vi "CODMn通讯.vi"() -> ()   [LabVIEW 2016, in "斯坦道CODMn新电路板.lvlib"]
uses:
  <vilib>/NI/Modbus Library/API/Wrapper/Create TCP Slave.vi
  <vilib>/Utility/config.llb/Write Key (String).vi
  <vilib>/Plasmionique/MB Master/MB_Master/MB_Master.lvclass
  <vilib>/NI/Modbus Library/API/slave/Modbus Slave.lvclass
  <vilib>/Utility/config.llb/NI_LVConfig.lvlib
  <vilib>/Plasmionique/MB Master/MB Master.lvlib
  <vilib>/NI/Modbus Library/API/Wrapper/API Main.lvlib
  Alarm interface/Alarm interface.lvlib
  <vilib>/ptbypt/NI_PtbyPt.lvlib
panel:
  out "控制命令 2":u16[](array[numeric]) format="%xH"
  out "状态告警区":T1 {"工作状态" items=["空闲"=0, "水样测试"=1, "标样核查"=2, "零点核查"=3, "跨度核查"=4, "空白测试"=5, "平行样测试"=6, "加标回收"=7, "空白校准"=8, "标样校准"=9, "初始化（清洗）"=10, "调试"=22, "填充管路"=30, "清洗管路"=31, "清洗反应杯"=32]; "告警代码" items=["无告警", "缺试剂告警", "缺水样告警", "缺蒸馏水告警", "缺标液告警", "仪表漏液告警", "标定异常告警", "超量程告警", "加热异常", "低试剂预警", "超上限告警", "超下限告警", "仪表内部其他异常", "滴定异常告警", "电极异常告警", "量程切换告警", "参数设置告警", "PH电极电位异常", "电导率电极异常", "浊度光度异常", "溶解氧电极异常", "溶解氧光强异常", "温度异常告警", "PH异常告警", "溶解氧异常告警", "电导率异常告警", "浊度异常告警", "叶绿素异常告警", "藻密度异常告警", "蓝绿藻异常告警", "ORP异常告警", "氨氮异常告警", "清洁刷异常告警", "SD卡异常告警", "蓝牙异常告警", "Wifi异常告警", "流程异常告警"]; "故障代码" items=["无故障", "电机故障", "温度故障", "通讯故障", "滴定故障"]}
  out "测量数据区":T2 {"单位" items=["ug/L", "mg/L", "ppm", "mg/m3", "cm", "ppb", "ug/m3", "%", "nmol/mol", "umol/mol", "MPN/L", "MPN/100ml", "ng/m3", "NTU", "无量纲", "ms/cm", "us/cm", "℃", "mV", "万个/L"]}
  out "状态告警区":u16[](array[numeric])
  out "测量数据区":u16[](array[numeric])
  out "序列号":string
  out "status":bool
  out "关键参数区":T3
  in  "读关键参数区":bool
  in  "读状态告警区":bool
  in  "读测量数据区":bool
  in  "站号":u16(ring) items=["CODMn"=21, "氨氮"=3]
  in  "停止":bool
  in  "启动":bool
  in  "控制命令":u16(ring) items=["启动测量"=1, "标样核查"=2, "零点核查"=3, "跨度核查"=4, "空白测试"=5, "平行样测试"=6, "加标回收"=7, "空白校准"=8, "标样校准"=9, "初始化（清洗）"=10, "停止测试"=11, "仪器重启"=12, "校时"=13, "模式设置"=14, "测量间隔设置"=15]
  in  "控制命令参数":u16[](array[numeric]) format="%04xH"
  in  "VISA Resource":refnum<visa-resource-name>
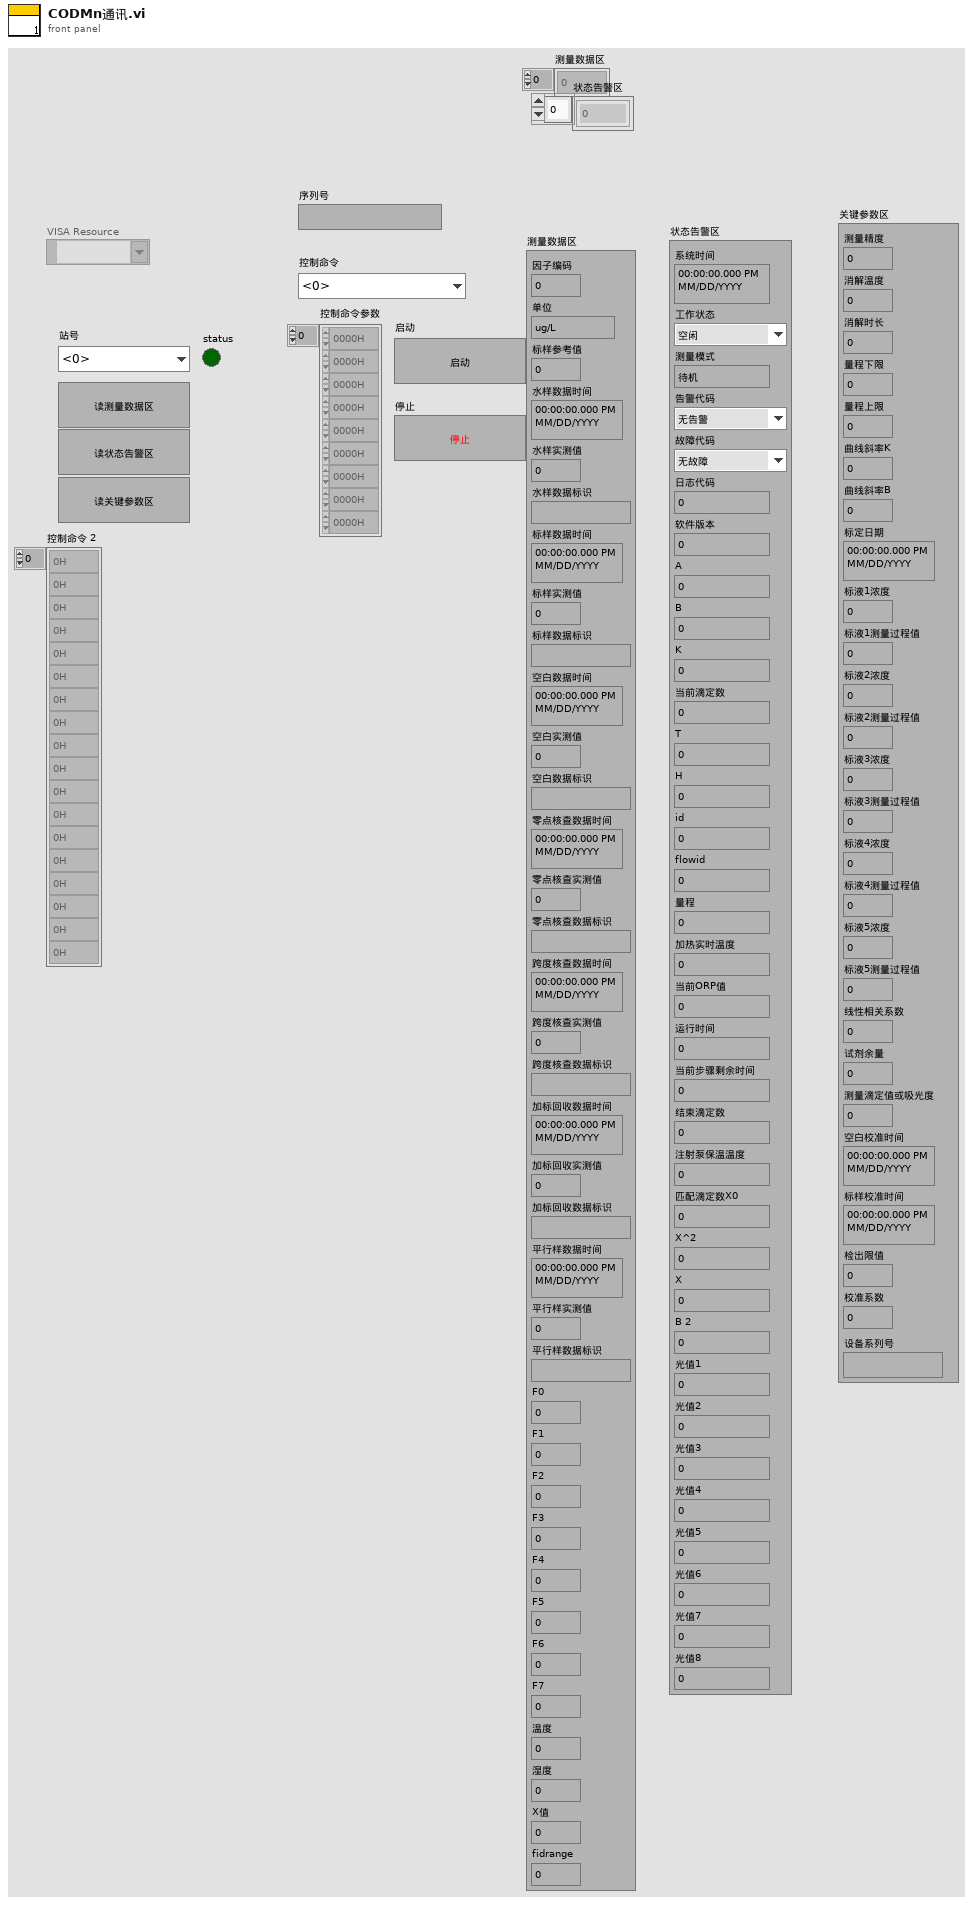
[diagram p1: front panel]
types:
  T1 = cluster{"系统时间":timestamp, "工作状态":u16, "测量模式":enum16{"待机", "连续模式", "周期模式", "定点模式", "受控模式", "手动模式"}, "告警代码":u16, "故障代码":u16, "日志代码":u16, "软件版本":u16, "A":sgl, "B":sgl, "K":sgl, "当前滴定数":sgl, "T":sgl, "H":sgl, "id":u16, "flowid":u16, "量程":u16, "加热实时温度":sgl, "当前ORP值":sgl, "运行时间":sgl, "当前步骤剩余时间":sgl, "结束滴定数":sgl, "注射泵保温温度":sgl, "匹配滴定数X0":u16, "X^2":sgl, "X":sgl, "B 2":sgl, "光值1":sgl, "光值2":sgl, "光值3":sgl, "光值4":sgl, "光值5":sgl, "光值6":sgl, "光值7":sgl, "光值8":sgl}
  T2 = cluster{"因子编码":u32, "单位":u16, "标样参考值":sgl, "水样数据时间":timestamp, "水样实测值":sgl, "水样数据标识":string, "标样数据时间":timestamp, "标样实测值":sgl, "标样数据标识":string, "空白数据时间":timestamp, "空白实测值":sgl, "空白数据标识":string, "零点核查数据时间":timestamp, "零点核查实测值":sgl, "零点核查数据标识":string, "跨度核查数据时间":timestamp, "跨度核查实测值":sgl, "跨度核查数据标识":string, "加标回收数据时间":timestamp, "加标回收实测值":sgl, "加标回收数据标识":string, "平行样数据时间":timestamp, "平行样实测值":sgl, "平行样数据标识":string, "F0":sgl, "F1":sgl, "F2":sgl, "F3":sgl, "F4":sgl, "F5":sgl, "F6":sgl, "F7":sgl, "温度":sgl, "湿度":sgl, "X值":sgl, "fidrange":sgl}
  T3 = cluster{"测量精度":u16, "消解温度":u16, "消解时长":u16, "量程下限":sgl, "量程上限":sgl, "曲线斜率K":sgl, "曲线斜率B":sgl, "标定日期":timestamp, "标液1浓度":sgl, "标液1测量过程值":sgl, "标液2浓度":sgl, "标液2测量过程值":sgl, "标液3浓度":sgl, "标液3测量过程值":sgl, "标液4浓度":sgl, "标液4测量过程值":sgl, "标液5浓度":sgl, "标液5测量过程值":sgl, "线性相关系数":sgl, "试剂余量":u32, "测量滴定值或吸光度":sgl, "空白校准时间":timestamp, "标样校准时间":timestamp, "检出限值":sgl, "校准系数":sgl, "设备系列号":string}
  T4 = enum16{"", "CODMn", "PH", "氨氮", "总氮", "总磷", "CODCr", "电导率", "水温", "溶解氧", "浊度", "叶绿素", "藻密度", "ORP"}
  T5 = typedef "CODMn交互.ctl" = cluster{"COD浓度（mg/L)":dbl, "水样启动时间":timestamp, "加标回收启动时间":timestamp, "CODMn工作状态":enum16{"空闲", "水样测试", "标样核查", "零点核查", "跨度核查", "空白测试", "平行样测试", "加标回收", "空白校准", "标样校准", "初始化（清洗）"}, "多列列表框":i32, "平台试剂余量百分比":sgl, "关键参数":cluster{"测量量程":dbl, "测量精度":dbl, "测量间隔":dbl, "消解温度":dbl, "消解时长":dbl, "空白校准时间":timestamp, "曲线截距":dbl, "曲线斜率":dbl, "测量检出限":dbl, "测量信号值":dbl, "线性相关系数":dbl, "二次多项式系数":dbl, "标样校准时间":timestamp, "稀释倍数":dbl, "三项式系数":dbl, "空白标定系数":dbl, "量程系数":dbl, "F0/ORPA":dbl, "F1/ORPB":dbl, "F2/ORPK":dbl, "F3":dbl, "F4":dbl, "F5":dbl, "F6":dbl, "F7":dbl, "X0/滴定数":dbl, "量程":dbl}, "关键参数改变":bool, "校准信息":cluster{"低标液1浓度":dbl, "低标液1信号值":dbl, "低标液1启用":u16, "低标液2浓度":dbl, "低标液2信号值":dbl, "低标液2启用":u16, "低标液3浓度":dbl, "低标液3信号值":dbl, "低标液3启用":u16, "低标液4浓度":dbl, "低标液4信号值":dbl, "低标液4启用":u16, "低标液5浓度":dbl, "低标液5信号值":dbl, "低标液5启用":u16, "高标液1浓度":dbl, "高标液1信号值":dbl, "高标液1启用":u16, "高标液2浓度":dbl, "高标液2信号值":dbl, "高标液2启用":u16, "高标液3浓度":dbl, "高标液3信号值":dbl, "高标液3启用":u16, "高标液4浓度":dbl, "高标液4信号值":dbl, "高标液4启用":u16, "高标液5浓度":dbl, "高标液5信号值":dbl, "高标液5启用":u16, "低斜率":dbl, "低截距":dbl, "低二次多项式系数":dbl, "低线性相关系数":dbl, "高斜率":dbl, "高截距":dbl, "高二次多项式系数":dbl, "高线性相关系数":dbl}, "校准信息改变":bool, "固件版本号":string}
  T6 = cluster{"测量模式":enum16{"水样测量", "标样核查", "零点核查", "跨度核查", "空白测试", "加标回收", "平行样", "校零", "校标"}}
  T7 = cluster{"时间标识":timestamp, "设备":string, "日志信息":string, "流程参数":string}
  T8 = typedef "NI_LVConfig.lvlib/Config Data RefNum.ctl" = refnum<k1>
  T9 = typedef "量程选择控件.ctl" = enum32{"L", "H", "AUTO"}
  T10 = cluster{"水样测试量程模式":T9, "标样核查量程模式":T9, "零点核查量程模式":T9, "跨度核查量程模式":T9, "空白测试量程模式":T9, "平行样测试量程模式":T9, "加标回收量程模式":T9, "空白校准量程模式":T9, "标样校准量程模式":T9}
  T11 = cluster{"测量量程":dbl, "测量精度":dbl, "测量间隔":dbl, "消解温度":dbl, "消解时长":dbl, "空白校准时间":timestamp, "曲线截距":dbl, "曲线斜率":dbl, "测量检出限":dbl, "测量信号值":dbl, "线性相关系数":dbl, "二次多项式系数":dbl, "标样校准时间":timestamp, "稀释倍数":dbl, "三项式系数":dbl, "空白标定系数":dbl, "量程系数":dbl, "F0/ORPA":dbl, "F1/ORPB":dbl, "F2/ORPK":dbl, "F3":dbl, "F4":dbl, "F5":dbl, "F6":dbl, "F7":dbl, "X0/滴定数":dbl, "量程":dbl}
  T12 = cluster{"低标液1浓度":dbl, "低标液1信号值":dbl, "低标液1启用":u16, "低标液2浓度":dbl, "低标液2信号值":dbl, "低标液2启用":u16, "低标液3浓度":dbl, "低标液3信号值":dbl, "低标液3启用":u16, "低标液4浓度":dbl, "低标液4信号值":dbl, "低标液4启用":u16, "低标液5浓度":dbl, "低标液5信号值":dbl, "低标液5启用":u16, "高标液1浓度":dbl, "高标液1信号值":dbl, "高标液1启用":u16, "高标液2浓度":dbl, "高标液2信号值":dbl, "高标液2启用":u16, "高标液3浓度":dbl, "高标液3信号值":dbl, "高标液3启用":u16, "高标液4浓度":dbl, "高标液4信号值":dbl, "高标液4启用":u16, "高标液5浓度":dbl, "高标液5信号值":dbl, "高标液5启用":u16, "低斜率":dbl, "低截距":dbl, "低二次多项式系数":dbl, "低线性相关系数":dbl, "高斜率":dbl, "高截距":dbl, "高二次多项式系数":dbl, "高线性相关系数":dbl}
  T13 = cluster{"站号":u16, "量程切换":enum32{"H", "L", "AUTO"}, "控制命令":u16, "模式设置":enum16{"待机", "连续模式", "周期模式", "定点模式", "受控模式", "手动模式"}, "测量间隔":u16}
  T14 = enum16{"水样测量", "标样核查", "零点核查", "跨度核查", "空白测试", "加标回收", "平行样", "校零", "校标"}
  T15 = enum8{"Enabled", "Disabled", "Disabled and Grayed Out"}
  T16 = typedef "Alarm interface.lvlib/map in.ctl" = cluster{"name":string, "CN":string, "FirmwareVersion":string, "code":string}
  T17 = typedef "工况数据.ctl" = cluster{"time":string, "data":cluster{"ups":cluster{"ups":cluster{"input_voltage":ext, "input_frequency":ext, "output_voltage":ext, "output_current":ext, "output_frequency":ext, "output_active_power":ext, "output_apparent_power":ext, "load_rate":ext, "cabinet_temperature":ext, "battery_voltage":ext, "remaining_battery_capacity":ext, "power_on_status":string, "power_supply_mode":string, "fault":bool, "battery_low_voltage":bool, "mains_supply_abnormality":bool}, "启用":bool}, "air_conditioner":cluster{"air_conditioner":cluster{"cabinet_temperature":ext, "air_supply_temperature":ext, "voltage":ext, "current":ext, "compressor_status":string, "Internal_fan_status":string, "external_fan_status":string, "heating_state":string, "refrigeration_state":bool, "high_temperature_alarm":bool, "low_temperature_alarm":bool, "heater_fault":bool, "temperature_sensor_fault":bool, "high_voltage_alarm":bool, "low_voltage_alarm":bool, "refrigeration_start_point":ext, "refrigeration_sensitive_point":ext, "heating_start_point":ext, "heating_sensitive_point":ext, "high_temperature_alarm_point":ext, "low_temperature_alarm_point":ext}, "启用":bool}, "smoke_sensor":cluster{"smoke_sensor":cluster{"trigger_alarm":bool}, "启用":bool}, "water_immersion_sensor":cluster{"water_immersion_sensor":cluster{"trigger_alarm":bool}, "启用":bool}, "temperature_and_humidity_sensor":cluster{"temperature_and_humidity_sensor":cluster{"current_temperature":ext, "current_humidity":ext, "room_temperature_alarm":bool, "humidity_alarm":bool}, "启用":bool}, "gps":cluster{"gps":cluster{"current_longitude":ext, "current_latitude":ext, "launch_longitude":ext, "launch_latitude":ext, "shift_alarm":bool}, "启用":bool}, "solar_controller":cluster{"solar_controller":cluster{"array_voltage":ext, "array_current":ext, "generating_power":ext, "battery_voltage":dbl, "battery_current":ext, "ceiling_voltage":ext, "minimum_voltage":ext, "battery_temperature":ext, "remaining_battery_capacity":ext, "load_voltage":ext, "load_current":ext, "load_power":ext, "equipment_temperature":ext, "accumulated_electricity_consumption_of_the_day":ext, "accumulated_electricity_consumption_of_the_current_month":ext, "accumulated_electricity_consumption_in_the_current_year":ext, "total_accumulated_power_consumption":ext, "accumulated_charging_capacity_of_the_day":ext, "accumulated_charging_amount_of_the_current_month":ext, "accumulated_charging_capacity_of_the_current_year":ext, "total_cumulative_charge":ext}, "启用":bool}, "solar_controller_2":cluster{"solar_controller_2":cluster{"array_voltage":ext, "array_current":ext, "generating_power":ext, "battery_voltage":dbl, "battery_current":ext, "ceiling_voltage":ext, "minimum_voltage":ext, "battery_temperature":ext, "remaining_battery_capacity":ext, "load_voltage":ext, "load_current":ext, "load_power":ext, "equipment_temperature":ext, "accumulated_electricity_consumption_of_the_day":ext, "accumulated_electricity_consumption_of_the_current_month":ext, "accumulated_electricity_consumption_in_the_current_year":ext, "total_accumulated_power_consumption":ext, "accumulated_charging_capacity_of_the_day":ext, "accumulated_charging_amount_of_the_current_month":ext, "accumulated_charging_capacity_of_the_current_year":ext, "total_cumulative_charge":ext}, "启用":bool}, "NH3":cluster{"NH3":cluster{"F0":ext, "F1":ext, "syringe_temperature":ext, "alarm_step":dbl, "X0":ext}, "启用":bool}, "TP":cluster{"TP":cluster{"F0":ext, "F1":ext, "F2":ext, "F3":ext, "digestion_temperature":ext, "constant_temperature":ext, "syringe_temperature":ext, "alarm_step":dbl, "X0":ext}, "启用":bool}, "TN":cluster{"TN":cluster{"F0":ext, "F1":ext, "F2":ext, "F3":ext, "F4":ext, "F5":ext, "F6":ext, "F7":ext, "digestion_temperature":ext, "constant_temperature":ext, "syringe_temperature":ext, "alarm_step":dbl, "X0":ext}, "启用":bool}, "CODMn":cluster{"CODMn":cluster{"temperature_curve":ext[], "titration_curve":ext[], "F0":ext, "F1":ext, "F2":ext, "F3":ext, "F4":ext, "F5":ext, "A":ext, "B":ext, "K":ext}, "启用":bool}, "CODCr":cluster{"CODCr":cluster{"temperature_curve":ext[], "F0":ext, "F1":ext, "reagent_sensor":ext}, "启用":bool}}}
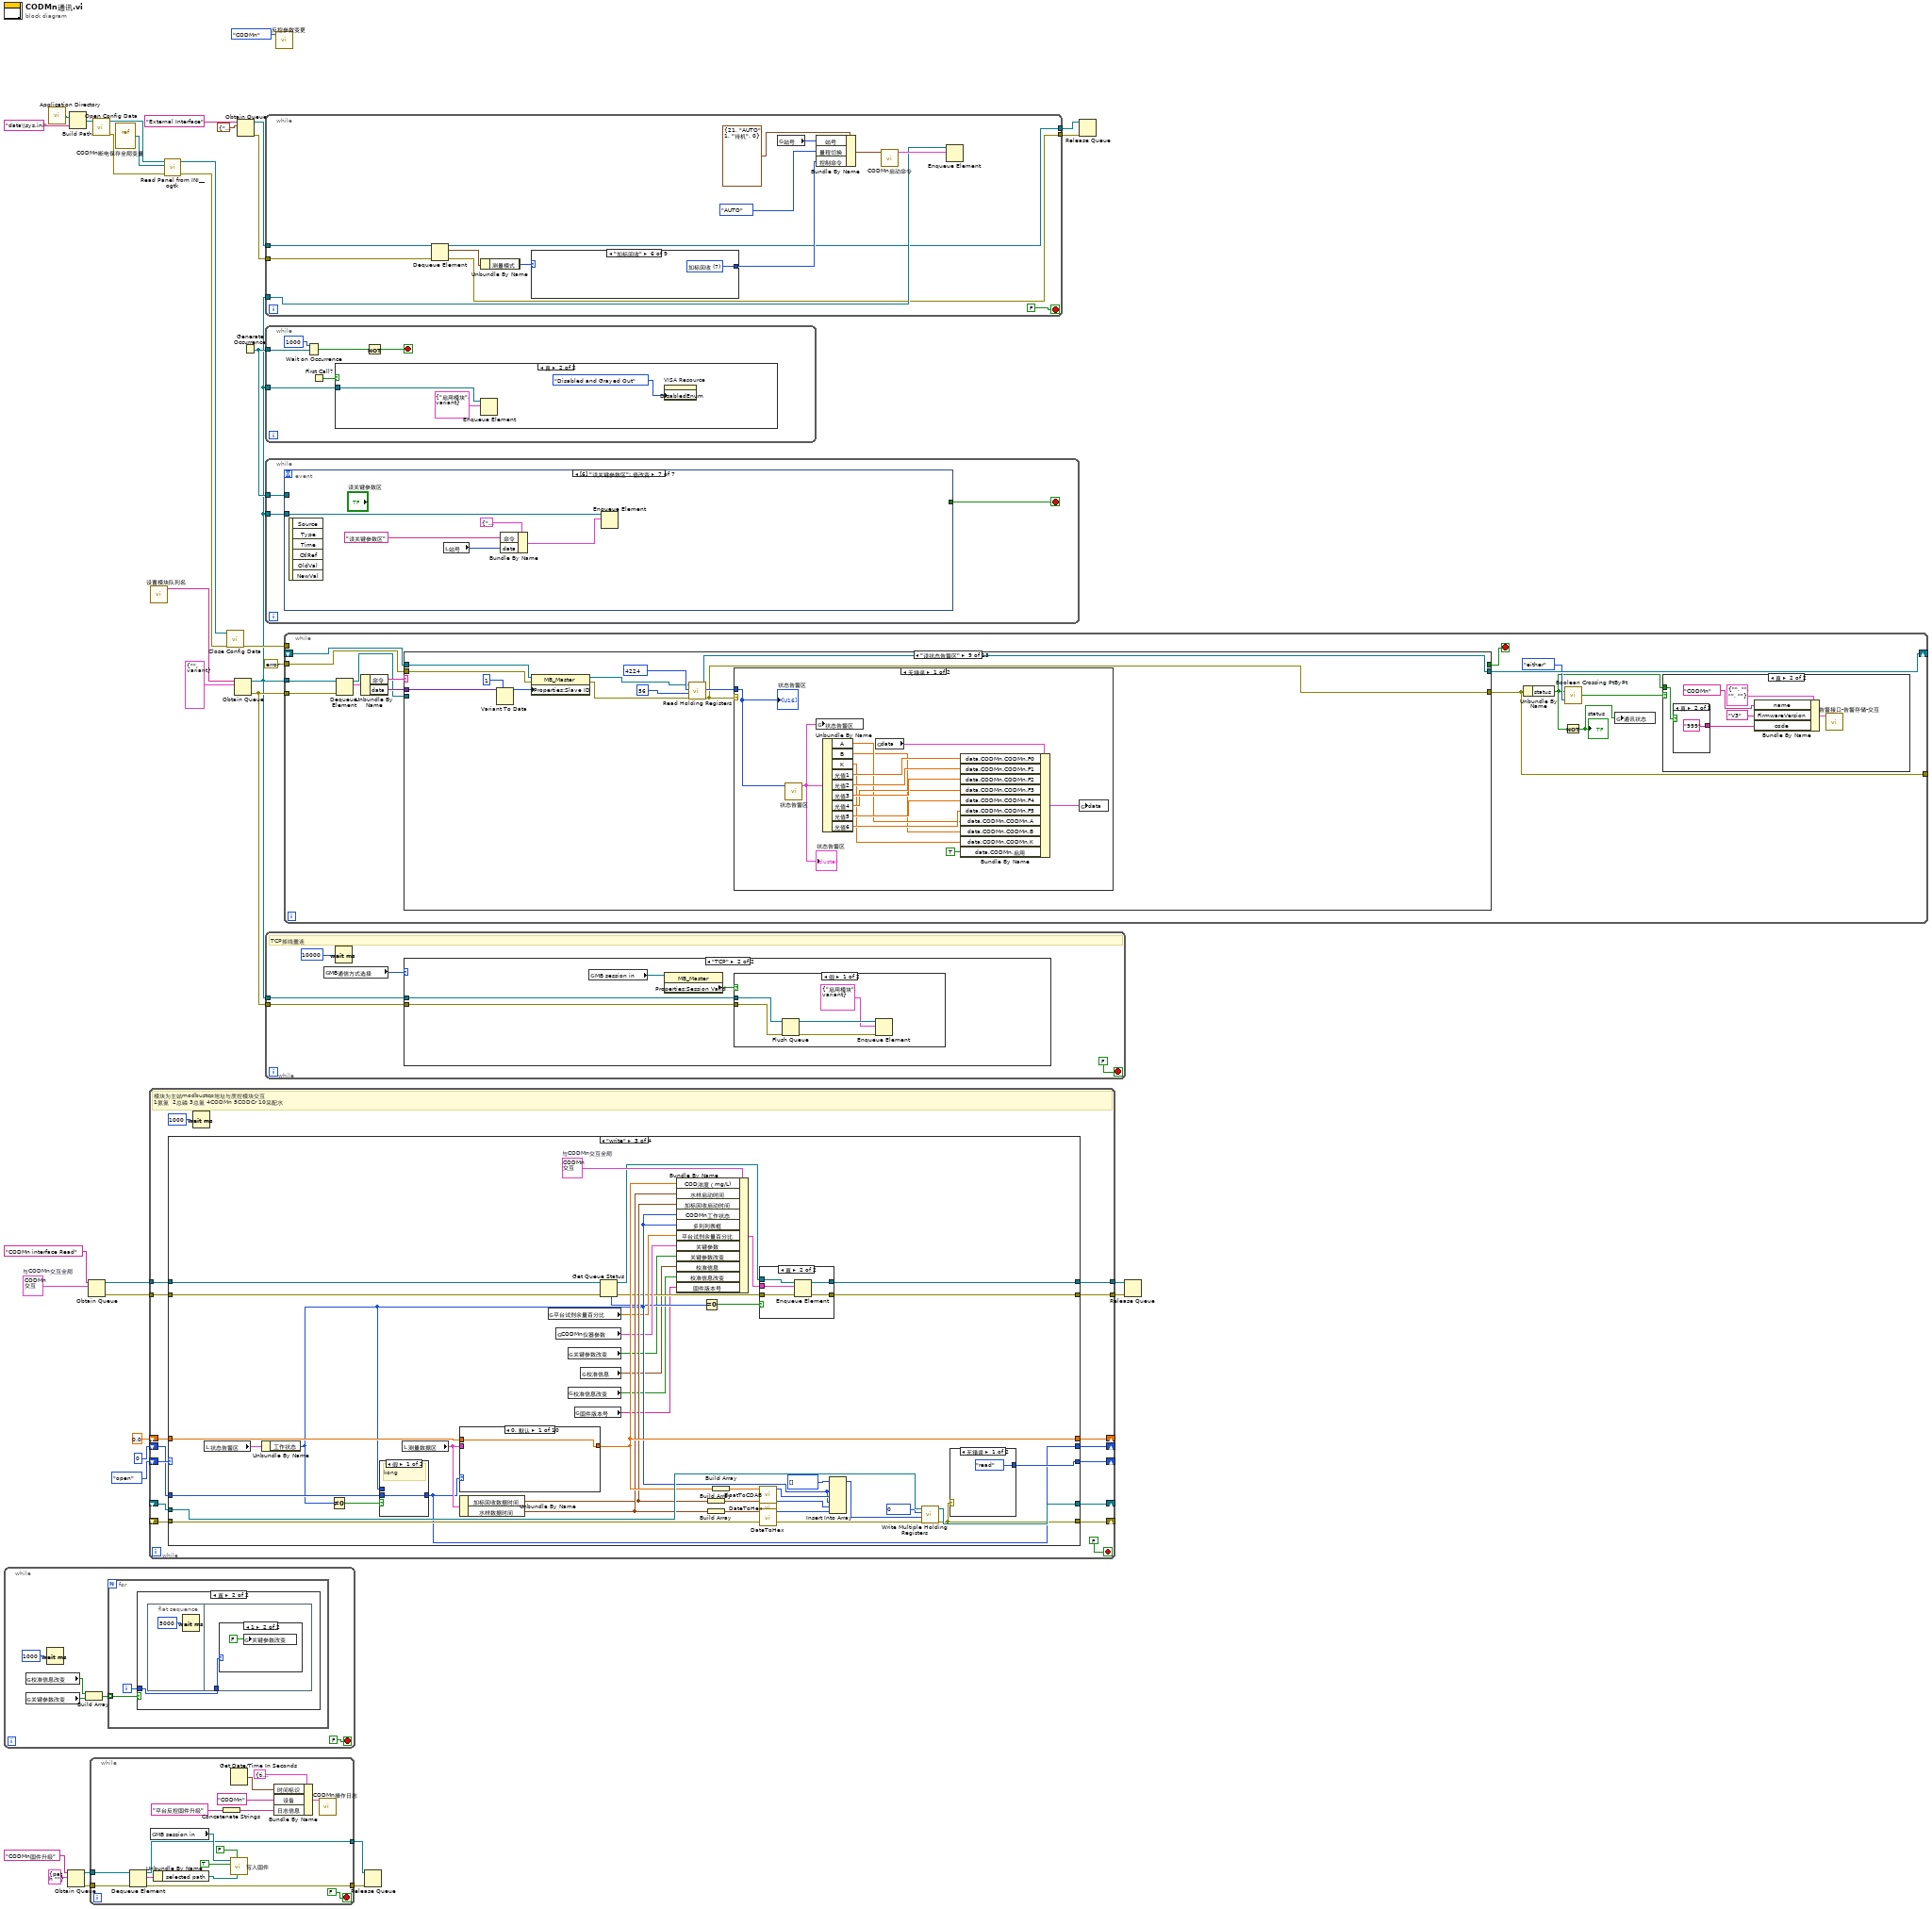
[diagram p0: block diagram]
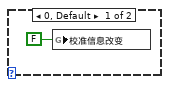
[diagram p3: hidden frame]
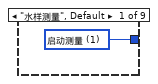
[diagram p4: hidden frame]
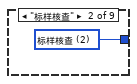
[diagram p5: hidden frame]
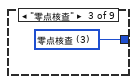
[diagram p6: hidden frame]
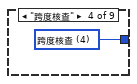
[diagram p7: hidden frame]
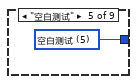
[diagram p8: hidden frame]
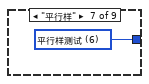
[diagram p9: hidden frame]
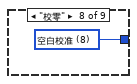
[diagram p10: hidden frame]
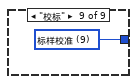
[diagram p11: hidden frame]
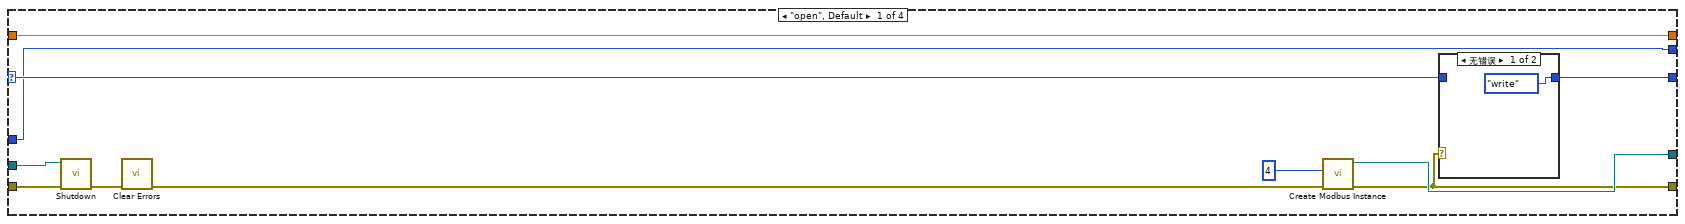
[diagram p14: hidden frame]
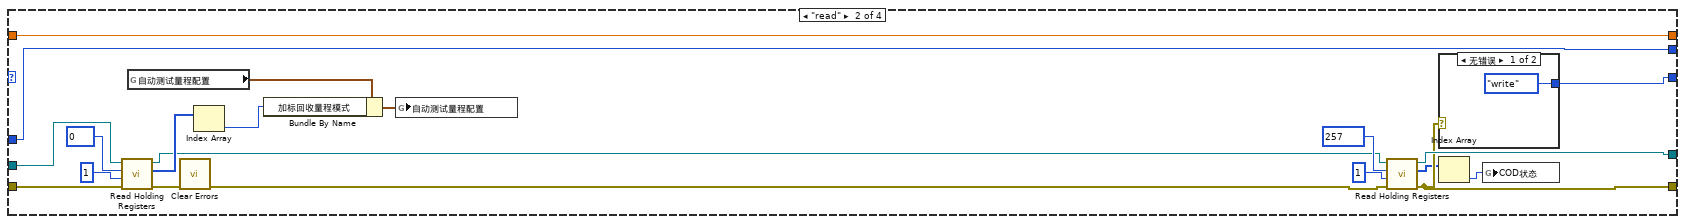
[diagram p16: hidden frame]
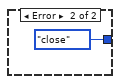
[diagram p17: hidden frame]
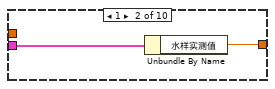
[diagram p20: hidden frame]
diagram:
  w14 = T5 {"COD浓度（mg/L)"=0.0, "水样启动时间"=timestamp(0 s since 1904-01-01), "加标回收启动时间"=timestamp(0 s since 1904-01-01), "CODMn工作状态"=enum."空闲", "多列列表框"=0, "平台试剂余量百分比"=0.0, "关键参数"={"测量量程"=0.0, "测量精度"=0.0, "测量间隔"=0.0, "消解温度"=0.0, "消解时长"=0.0, "空白校准时间"=timestamp(0 s since 1904-01-01), "曲线截距"=0.0, "曲线斜率"=0.0, "测量检出限"=0.0, "测量信号值"=0.0, "线性相关系数"=0.0, "二次多项式系数"=0.0, "标样校准时间"=timestamp(0 s since 1904-01-01), "稀释倍数"=0.0, "三项式系数"=0.0, "空白标定系数"=0.0, "量程系数"=0.0, "F0/ORPA"=0.0, "F1/ORPB"=0.0, "F2/ORPK"=0.0, "F3"=0.0, "F4"=0.0, "F5"=0.0, "F6"=0.0, "F7"=0.0, "X0/滴定数"=0.0, "量程"=0.0}, "关键参数改变"=FALSE, "校准信息"={"低标液1浓度"=0.0, "低标液1信号值"=0.0, "低标液1启用"=0, "低标液2浓度"=0.0, "低标液2信号值"=0.0, "低标液2启用"=0, "低标液3浓度"=0.0, "低标液3信号值"=0.0, "低标液3启用"=0, "低标液4浓度"=0.0, "低标液4信号值"=0.0, "低标液4启用"=0, "低标液5浓度"=0.0, "低标液5信号值"=0.0, "低标液5启用"=0, "高标液1浓度"=0.0, "高标液1信号值"=0.0, "高标液1启用"=0, "高标液2浓度"=0.0, "高标液2信号值"=0.0, "高标液2启用"=0, "高标液3浓度"=0.0, "高标液3信号值"=0.0, "高标液3启用"=0, "高标液4浓度"=0.0, "高标液4信号值"=0.0, "高标液4启用"=0, "高标液5浓度"=0.0, "高标液5信号值"=0.0, "高标液5启用"=0, "低斜率"=0.0, "低截距"=0.0, "低二次多项式系数"=0.0, "低线性相关系数"=0.0, "高斜率"=0.0, "高截距"=0.0, "高二次多项式系数"=0.0, "高线性相关系数"=0.0}, "校准信息改变"=FALSE, "固件版本号"=""}  # 与CODMn交互全局
  n1 = while {
    stop <- FALSE stop-if-true
    n2 = global read "CODMn断电保存全局变量.vi" "校准信息改变"() -> (w40:bool)
    n3 = global read "CODMn断电保存全局变量.vi" "关键参数改变"() -> (w39:bool)
    n4 = Wait (ms)(milliseconds to wait=u32 1000 ("等待时间（毫秒）")) -> ()  [unwired: 1 out]
    n5 = Build Array(w40, w39) -> (w38:bool[])
    n6 = for {
      tunnel: w38 -> [w44] mode=indexing
      i -> [w43]
      n7 = case shown="真" w44 {
        tunnel: w43 -> [_ w45]
        frame False {
        }
        frame True {
          n8 = flat-sequence {
            tunnel: w45 -> [w47]
            frame #0 {
              n9 = Wait (ms)(milliseconds to wait=u32 5000 ("等待时间（毫秒）")) -> ()  [unwired: 1 out]
            }
            frame #1 {
              n10 = case shown="1" w47 {
                frame 0, Default {
                  n11 = global write "CODMn断电保存全局变量.vi" "校准信息改变"(FALSE ("关键参数改变")) -> ()
                }
                frame 1 {
                  n12 = global write "CODMn断电保存全局变量.vi" "关键参数改变"(FALSE ("关键参数改变")) -> ()
                }
              }
            }
          }
        }
      }
    }
  }
  n13 = call <vilib>:"Application Directory.vi"() -> ("Application Directory"=w9:path)
  n14 = Obtain Queue(name (unnamed)="CODMn固件升级" ("名称（未命名）"), element data type=cluster{"selected path":path} {"selected path"=path ""}) -> (queue out=w5:refnum<queue>, error out=w4:errorcluster)  [unwired: 3 in, 1 out]
  n15 = Build Path(base path=w9, name or relative path="data\\sys.ini" ("名称或相对路径")) -> (appended path=w26:path)
  n16 = Obtain Queue(name (unnamed)="CODMn interface Read" ("写入方名称"), element data type=w14) -> (queue out=w16:refnum<queue>, error out=w11:errorcluster)  [unwired: 3 in, 1 out]
  n17 = while {
    tunnel: w5 -> [w63]
    tunnel: w4 -> [w62]
    tunnel: [w58] -> w3
    tunnel: [w57] -> w2
    stop <- FALSE stop-if-true
    n18 = Dequeue Element(queue=w63, error in (no error)=w62) -> (queue out=w58:refnum<queue>, element=w61:cluster{"selected path":path}, error out=w57:errorcluster)  [unwired: 1 in, 1 out]
    n19 = global read "VARCODMn全局变量.vi" "MB session in"() -> (w65:refnum<class "MB_Master.lvclass">)
    n20 = Unbundle By Name(w61) -> ("selected path"=w60:path)
    n21 = Concatenate Strings("平台反控固件升级" ("日志信息")) -> (w50:string)
    n22 = Get Date/Time In Seconds() -> (seconds since 1Jan1904=w52:timestamp)
    n23 = call "写入固件.vi"("selected path"=w60, "路径对话框"=FALSE, "保留原配置"=TRUE, "MB session in"=w65) -> ()  [unwired: 6 in, 2 out]
    n24 = Bundle By Name(cluster=T7 {"时间标识"=timestamp(0 s since 1904-01-01), "设备"="", "日志信息"="", "流程参数"=""} ("data in"), "时间标识"=w52, "设备"="CODMn", "日志信息"=w50) -> (w54:T7)
    n25 = call "CODMn操作日志.vi"("data in"=w54) -> ()  [unwired: 11 in]
  }
  n26 = call <vilib>:"Open Config Data.vi"("configuration file path"=w26) -> ("error out"=w33:errorcluster, "refnum"=w30:T8)  [unwired: 8 in, 1 out]
  n27 = vi-ref "CODMn断电保存全局变量.vi"() -> (w31:refnum<vi>)
  n28 = while {
    shift-right: [w79] -> _
    shift-left: _ -> [w81]
    shift-right: [w78] -> _
    shift-left: _ -> [w80]
    shift-right: [w75] -> _
    shift-left: enum16{"open", "read", "write", "close"}."open" -> [w76]
    shift-right: [w73] -> _
    shift-left: sgl 0.0 ("标样实测值") -> [w72]
    shift-right: [w71] -> _
    shift-left: u16 0 ("工作状态") -> [w70]
    tunnel: w16 -> [w69]
    tunnel: [w68] -> w13
    tunnel: [w67] -> w12
    tunnel: w11 -> [w66]
    stop <- FALSE stop-if-true
    # "模块为主站modbustcp地址与质控模块交互\n1氨氮  2总磷 3总氮 4CODMn 5CODCr 10采配水"
    n29 = case shown="\"write\"" w76 {
      selector: w76 -> [w92 _ _ _]
      tunnel: w81 -> [w86 w102 w155 w191]
      tunnel: w80 -> [w85 w101 w154 w190]
      tunnel: [w89 w113 w152 w191] -> w79
      tunnel: [w88 w112 w151 w193] -> w78
      tunnel: [w91 w114 w156 enum16{"open", "read", "write", "close"}."open"] -> w75
      tunnel: [w83 w107 w135 w188] -> w73
      tunnel: w72 -> [w83 w107 w148 w188]
      tunnel: [w82 w106 w139 w187] -> w71
      tunnel: w70 -> [w82 w106 w138 w187]
      tunnel: w69 -> [_ _ w129 _]
      tunnel: [_ _ w127 _] -> w68
      tunnel: [_ _ w126 _] -> w67
      tunnel: w66 -> [_ _ w122 _]
      frame "open", Default {
        n30 = call-dynamic "Shutdown.vi"("error in"=w85, "Modbus slave in"=w86) -> ("error out"=w84:errorcluster)  [unwired: 9 in]
        n31 = call <vilib>:"Clear Errors.vi"("error in (no error)"=w84) -> ("error out"=w87:errorcluster)  [unwired: 5 in, 1 out]
        n32 = call-poly <vilib>:"Create Modbus Instance.vi"("error in"=w87, "port (502)"=u16 4) -> ("error out"=w88:errorcluster, "TCP slave instance"=w89:refnum<class "Modbus Slave.lvclass">)  [unwired: 8 in]
        n33 = case shown="无错误" w88 {
          tunnel: w92 -> [_ w94]
          tunnel: [enum16{"open", "read", "write", "close"}."write" w94] -> w91
          frame No Error {
          }
          frame Error {
          }
        }
      }
      frame "read" {
        n34 = call-dynamic <vilib>:"Read Holding Registers.vi"("error in"=w101, "number of inputs"=u16 1, "starting address"=u16 0, "Modbus slave in"=w102) -> ("error out"=w100:errorcluster, "register values"=w105:u16[], "Modbus slave out"=w99:refnum<class "Modbus Slave.lvclass">)  [unwired: 5 in]
        n35 = global read "CODMn断电保存全局变量.vi" "自动测试量程配置"() -> (w97:T10)
        n36 = call <vilib>:"Clear Errors.vi"("error in (no error)"=w100) -> ("error out"=w95:errorcluster)  [unwired: 5 in, 1 out]
        n37 = Index Array(array=w105) -> (element=w96:u16)  [unwired: 1 in]
        n38 = Bundle By Name(cluster=w97, "加标回收量程模式"=w96) -> (w98:T10)
        n39 = global write "CODMn断电保存全局变量.vi" "自动测试量程配置"(w98) -> ()
        n40 = call-dynamic <vilib>:"Read Holding Registers.vi"("error in"=w95, "number of inputs"=u16 1, "starting address"=u16 257, "Modbus slave in"=w99) -> ("error out"=w112:errorcluster, "register values"=w109:u16[], "Modbus slave out"=w113:refnum<class "Modbus Slave.lvclass">)  [unwired: 5 in]
        n41 = case shown="无错误" w112 {
          tunnel: [enum16{"open", "read", "write", "close"}."write" enum16{"open", "read", "write", "close"}."close"] -> w114
          frame No Error {
          }
          frame Error {
          }
        }
        n42 = Index Array(array=w109) -> (element=w108:u16)  [unwired: 1 in]
        n43 = global write "VARCODMn全局变量.vi" "COD状态"(w108) -> ()
      }
      frame "write" {
        w136 = T5 {"COD浓度（mg/L)"=0.0, "水样启动时间"=timestamp(0 s since 1904-01-01), "加标回收启动时间"=timestamp(0 s since 1904-01-01), "CODMn工作状态"=enum."空闲", "多列列表框"=0, "平台试剂余量百分比"=0.0, "关键参数"={"测量量程"=0.0, "测量精度"=0.0, "测量间隔"=0.0, "消解温度"=0.0, "消解时长"=0.0, "空白校准时间"=timestamp(0 s since 1904-01-01), "曲线截距"=0.0, "曲线斜率"=0.0, "测量检出限"=0.0, "测量信号值"=0.0, "线性相关系数"=0.0, "二次多项式系数"=0.0, "标样校准时间"=timestamp(0 s since 1904-01-01), "稀释倍数"=0.0, "三项式系数"=0.0, "空白标定系数"=0.0, "量程系数"=0.0, "F0/ORPA"=0.0, "F1/ORPB"=0.0, "F2/ORPK"=0.0, "F3"=0.0, "F4"=0.0, "F5"=0.0, "F6"=0.0, "F7"=0.0, "X0/滴定数"=0.0, "量程"=0.0}, "关键参数改变"=FALSE, "校准信息"={"低标液1浓度"=0.0, "低标液1信号值"=0.0, "低标液1启用"=0, "低标液2浓度"=0.0, "低标液2信号值"=0.0, "低标液2启用"=0, "低标液3浓度"=0.0, "低标液3信号值"=0.0, "低标液3启用"=0, "低标液4浓度"=0.0, "低标液4信号值"=0.0, "低标液4启用"=0, "低标液5浓度"=0.0, "低标液5信号值"=0.0, "低标液5启用"=0, "高标液1浓度"=0.0, "高标液1信号值"=0.0, "高标液1启用"=0, "高标液2浓度"=0.0, "高标液2信号值"=0.0, "高标液2启用"=0, "高标液3浓度"=0.0, "高标液3信号值"=0.0, "高标液3启用"=0, "高标液4浓度"=0.0, "高标液4信号值"=0.0, "高标液4启用"=0, "高标液5浓度"=0.0, "高标液5信号值"=0.0, "高标液5启用"=0, "低斜率"=0.0, "低截距"=0.0, "低二次多项式系数"=0.0, "低线性相关系数"=0.0, "高斜率"=0.0, "高截距"=0.0, "高二次多项式系数"=0.0, "高线性相关系数"=0.0}, "校准信息改变"=FALSE, "固件版本号"=""}  # 与CODMn交互全局
        n44 = local read "状态告警区"() -> (w137:T1)
        n45 = Unbundle By Name(w137) -> ("工作状态"=w132:u16)
        n46 = Not Equal To 0?(x=w132) -> (x != 0?=w140:bool)
        n47 = case shown="假" w140 {
          tunnel: w132 -> [_ w165]
          tunnel: [w164 w165] -> w139
          tunnel: w138 -> [w164 _]
          frame False {
            # "kong"
          }
          frame True {
            # "..."
          }
        }
        n48 = local read "测量数据区"() -> (w145:T2)
        n49 = case shown="0, 默认" w139 {
          tunnel: [w166 w168 w170 w172 w174 w176 w178 w180 w182 w184] -> w135
          tunnel: w148 -> [w166 _ _ _ _ _ _ _ _ _]
          tunnel: w145 -> [_ w167 w169 w171 w173 w175 w177 w179 w181 w183]
          frame 0, Default {
          }
          frame 1 {
            n50 = Unbundle By Name(w167) -> ("水样实测值"=w168:sgl)
          }
          frame 2 {
            n51 = Unbundle By Name(w169) -> ("标样实测值"=w170:sgl)
          }
          frame 3 {
            n52 = Unbundle By Name(w171) -> ("零点核查实测值"=w172:sgl)
          }
          frame 4 {
            n53 = Unbundle By Name(w173) -> ("跨度核查实测值"=w174:sgl)
          }
          frame 5 {
            n54 = Unbundle By Name(w175) -> ("空白实测值"=w176:sgl)
          }
          frame 6 {
            n55 = Unbundle By Name(w177) -> ("平行样实测值"=w178:sgl)
          }
          frame 7 {
            n56 = Unbundle By Name(w179) -> ("加标回收实测值"=w180:sgl)
          }
          frame 8 {
            n57 = Unbundle By Name(w181) -> ("空白实测值"=w182:sgl)
          }
          frame 9 {
            n58 = Unbundle By Name(w183) -> ("标样实测值"=w184:sgl)
          }
        }
        n59 = Unbundle By Name(w145) -> ("加标回收数据时间"=w133:timestamp, "水样数据时间"=w134:timestamp)
        n60 = global read "VARCODMn全局变量.vi" "平台试剂余量百分比"() -> (w131:sgl)
        n61 = global read "CODMn断电保存全局变量.vi" "CODMn仪器参数"() -> (w130:T11)
        n62 = global read "CODMn断电保存全局变量.vi" "关键参数改变"() -> (w120:bool)
        n63 = global read "CODMn断电保存全局变量.vi" "校准信息改变"() -> (w118:bool)
        n64 = global read "VARCODMn全局变量.vi" "固件版本号"() -> (w117:string)
        n65 = global read "CODMn断电保存全局变量.vi" "校准信息"() -> (w119:T12)
        n66 = Get Queue Status(queue=w129, error in (no error)=w122) -> (queue out=w125:refnum<queue>, error out=w121:errorcluster, # elements in queue=w124:i32)  [unwired: 1 in, 5 out]
        n67 = Bundle By Name(cluster=w136, "COD浓度（mg/L)"=w135, "水样启动时间"=w134, "加标回收启动时间"=w133, "CODMn工作状态"=w132, "多列列表框"=w132, "平台试剂余量百分比"=w131, "关键参数"=w130, "关键参数改变"=w120, "校准信息"=w119, "校准信息改变"=w118, "固件版本号"=w117) -> (w128:T5)
        n68 = Equal To 0?(x=w124) -> (x = 0?=w123:bool)
        n69 = Build Array(w133) -> (w144:timestamp[])
        n70 = Build Array(w134) -> (w142:timestamp[])
        n71 = Build Array(w135) -> (w147:sgl[])
        n72 = case shown="真" w123 {
          tunnel: w125 -> [w158 w163]
          tunnel: w128 -> [_ w162]
          tunnel: [w158 w161] -> w127
          tunnel: [w157 w160] -> w126
          tunnel: w121 -> [w157 w159]
          frame False {
          }
          frame True {
            n73 = Enqueue Element(queue=w163, element=w162, error in (no error)=w159) -> (queue out=w161:refnum<queue>, error out=w160:errorcluster)  [unwired: 1 in, 1 out]
          }
        }
        n74 = call "FloatToCDAB.vi"("浮点数"=w147) -> ("CDAB整形输出"=w146:u16[])  [unwired: 10 in]
        n75 = call "DateToHex.vi"("DATE"=w144) -> ("数组"=w143:u16[])  [unwired: 10 in]
        n76 = call "DateToHex.vi"("DATE"=w142) -> ("数组"=w141:u16[])  [unwired: 10 in]
        n77 = Insert Into Array(array=u16[] [] ("values"), new element #1=w132, new element #2=w146, new element #3=w132, new element #4=w143, new element #5=w141) -> (w149:u16[])  [unwired: 1 in]
        n78 = call-dynamic "Write Multiple Holding Registers.vi"("error in"=w154, "registers to write"=w149, "starting address"=u16 0, "Modbus slave in"=w155) -> ("error out"=w151:errorcluster, "Modbus slave out"=w152:refnum<class "Modbus Slave.lvclass">)  [unwired: 6 in]
        n79 = case shown="无错误" w151 {
          tunnel: [enum16{"open", "read", "write", "close"}."read" enum16{"open", "read", "write", "close"}."close"] -> w156
          frame No Error {
          }
          frame Error {
          }
        }
      }
      frame "close" {
        n80 = call-dynamic "Shutdown.vi"("error in"=w190, "Modbus slave in"=w191) -> ("error out"=w189:errorcluster)  [unwired: 9 in]
        n81 = call <vilib>:"Clear Errors.vi"("error in (no error)"=w189) -> ("error out"=w193:errorcluster)  [unwired: 5 in, 1 out]
      }
    }
    n82 = Wait (ms)(milliseconds to wait=u32 1000 ("等待时间（毫秒）")) -> ()  [unwired: 1 out]
  }
  n83 = call "设置模块队列名.vi"() -> ("Msg"=w10:string)  [unwired: 11 in]
  n84 = call <userlib>:"Read Panel from INI__ogtk.vi"("error in (no error)"=w33, "VI ref"=w31, "refnum"=w30) -> ("error out"=w34:errorcluster, "refnum out"=w32:T8)  [unwired: 7 in]
  n85 = call <vilib>:"Close Config Data.vi"("error in (no error)"=w34, "refnum"=w32) -> ("error out"=w29:errorcluster)  [unwired: 8 in, 1 out]
  n86 = Obtain Queue(name (unnamed)=w10, element data type=cluster{"命令":string, "data":variant} {"命令"="", "data"=variant}) -> (queue out=w21:refnum<queue>, error out=w27:errorcluster)  [unwired: 3 in, 1 out]
  n87 = Obtain Queue(name (unnamed)="External Interface" ("名称（未命名）"), element data type=T6 {"测量模式"=enum."水样测量"} ("元素")) -> (queue out=w23:refnum<queue>, error out=w22:errorcluster)  [unwired: 3 in, 1 out]
  n88 = Generate Occurrence() -> (w35:refnum<k4>)
  n89 = while {
    tunnel: w23 -> [w207]
    tunnel: w22 -> [w206]
    tunnel: w21 -> [w198]
    tunnel: [w197] -> w20
    tunnel: [w196] -> w19
    stop <- FALSE stop-if-true
    n90 = Dequeue Element(queue=w207, error in (no error)=w206) -> (queue out=w197:refnum<queue>, element=w201:T6, error out=w196:errorcluster)  [unwired: 1 in, 1 out]
    n91 = Unbundle By Name(w201) -> ("测量模式"=w200:T14)
    n92 = case shown="\"加标回收\"" w200 {
      tunnel: [w208 w209 w210 w211 w212 w213 w214 w215 w216] -> w199
      frame "水样测量", Default {
        w208 = u16 1 items=["启动测量"=1, "标样核查"=2, "零点核查"=3, "跨度核查"=4, "空白测试"=5, "平行样测试"=6, "加标回收"=7, "空白校准"=8, "标样校准"=9, "初始化（清洗）"=10, "停止测试"=11, "仪器重启"=12, "校时"=13, "模式设置"=14, "测量间隔设置"=15, "调试"=22, "填充管路"=30, "清洗管路"=31, "清洗反应杯"=32] ("控制命令")
      }
      frame "标样核查" {
        w209 = u16 2 items=["启动测量"=1, "标样核查"=2, "零点核查"=3, "跨度核查"=4, "空白测试"=5, "平行样测试"=6, "加标回收"=7, "空白校准"=8, "标样校准"=9, "初始化（清洗）"=10, "停止测试"=11, "仪器重启"=12, "校时"=13, "模式设置"=14, "测量间隔设置"=15, "调试"=22, "填充管路"=30, "清洗管路"=31, "清洗反应杯"=32] ("控制命令")
      }
      frame "零点核查" {
        w210 = u16 3 items=["启动测量"=1, "标样核查"=2, "零点核查"=3, "跨度核查"=4, "空白测试"=5, "平行样测试"=6, "加标回收"=7, "空白校准"=8, "标样校准"=9, "初始化（清洗）"=10, "停止测试"=11, "仪器重启"=12, "校时"=13, "模式设置"=14, "测量间隔设置"=15, "调试"=22, "填充管路"=30, "清洗管路"=31, "清洗反应杯"=32] ("控制命令")
      }
      frame "跨度核查" {
        w211 = u16 4 items=["启动测量"=1, "标样核查"=2, "零点核查"=3, "跨度核查"=4, "空白测试"=5, "平行样测试"=6, "加标回收"=7, "空白校准"=8, "标样校准"=9, "初始化（清洗）"=10, "停止测试"=11, "仪器重启"=12, "校时"=13, "模式设置"=14, "测量间隔设置"=15, "调试"=22, "填充管路"=30, "清洗管路"=31, "清洗反应杯"=32] ("控制命令")
      }
      frame "空白测试" {
        w212 = u16 5 items=["启动测量"=1, "标样核查"=2, "零点核查"=3, "跨度核查"=4, "空白测试"=5, "平行样测试"=6, "加标回收"=7, "空白校准"=8, "标样校准"=9, "初始化（清洗）"=10, "停止测试"=11, "仪器重启"=12, "校时"=13, "模式设置"=14, "测量间隔设置"=15, "调试"=22, "填充管路"=30, "清洗管路"=31, "清洗反应杯"=32] ("控制命令")
      }
      frame "加标回收" {
        w213 = u16 7 items=["启动测量"=1, "标样核查"=2, "零点核查"=3, "跨度核查"=4, "空白测试"=5, "平行样测试"=6, "加标回收"=7, "空白校准"=8, "标样校准"=9, "初始化（清洗）"=10, "停止测试"=11, "仪器重启"=12, "校时"=13, "模式设置"=14, "测量间隔设置"=15, "调试"=22, "填充管路"=30, "清洗管路"=31, "清洗反应杯"=32] ("控制命令")
      }
      frame "平行样" {
        w214 = u16 6 items=["启动测量"=1, "标样核查"=2, "零点核查"=3, "跨度核查"=4, "空白测试"=5, "平行样测试"=6, "加标回收"=7, "空白校准"=8, "标样校准"=9, "初始化（清洗）"=10, "停止测试"=11, "仪器重启"=12, "校时"=13, "模式设置"=14, "测量间隔设置"=15, "调试"=22, "填充管路"=30, "清洗管路"=31, "清洗反应杯"=32] ("控制命令")
      }
      frame "校零" {
        w215 = u16 8 items=["启动测量"=1, "标样核查"=2, "零点核查"=3, "跨度核查"=4, "空白测试"=5, "平行样测试"=6, "加标回收"=7, "空白校准"=8, "标样校准"=9, "初始化（清洗）"=10, "停止测试"=11, "仪器重启"=12, "校时"=13, "模式设置"=14, "测量间隔设置"=15, "调试"=22, "填充管路"=30, "清洗管路"=31, "清洗反应杯"=32] ("控制命令")
      }
      frame "校标" {
        w216 = u16 9 items=["启动测量"=1, "标样核查"=2, "零点核查"=3, "跨度核查"=4, "空白测试"=5, "平行样测试"=6, "加标回收"=7, "空白校准"=8, "标样校准"=9, "初始化（清洗）"=10, "停止测试"=11, "仪器重启"=12, "校时"=13, "模式设置"=14, "测量间隔设置"=15, "调试"=22, "填充管路"=30, "清洗管路"=31, "清洗反应杯"=32] ("控制命令")
      }
    }
    n93 = global read "CODMn断电保存全局变量.vi" "站号"() -> (w202:u16)
    n94 = Bundle By Name(cluster=T13 {"站号"=21, "量程切换"=enum."AUTO", "控制命令"=1, "模式设置"=enum."待机", "测量间隔"=0} ("参数"), "站号"=w202, "量程切换"=enum32{"H", "L", "AUTO"}."AUTO", "控制命令"=w199) -> (w203:T13)
    n95 = call "CODMn启动命令.vi"("参数"=w203) -> ("启动命令"=w205:cluster{"命令":string, "data":variant})  [unwired: 10 in]
    n96 = Enqueue Element(queue=w198, element=w205) -> ()  [unwired: 2 in, 3 out]
  }
  n97 = while {
    tunnel: w35 -> [w222]
    tunnel: w21 -> [w218]
    stop <- w219 stop-if-true
    n98 = Wait on Occurrence(2:w222, 3:1000 ("毫秒超时(-1)")) -> (0:w220:bool)  [unwired: 1 in]
    n99 = First Call?() -> (First Call?: T/F=w217:bool)
    n100 = case shown="真" w217 {
      tunnel: w218 -> [_ w224]
      frame False {
      }
      frame True {
        n101 = Enqueue Element(queue=w224, element=cluster{"命令":string, "data":variant} {"命令"="启用模块", "data"=variant} ("元素")) -> ()  [unwired: 2 in, 3 out]
        n102 = property on="VISA Resource" class="VISAName"("DisabledEnum"=T15."Disabled and Grayed Out" ("禁用")) -> ()  [unwired: 2 in, 2 out]
      }
    }
    n103 = Not(x=w220) -> (.not. x?=w219:bool)
  }
  n104 = while {
    tunnel: w21 -> [w228]
    tunnel: w35 -> [w226]
    stop <- w227 stop-if-true
    n105 = event shown="[6] \"读关键参数区\": 值改变" {
      selector: _ -> [_ _ _ _ _ _ _]
      dyn-events: _ -> [_ _ _ _ _ _ _]
      timeout: _ -> [_ _ _ _ _ _ _]
      tunnel: w228 -> [_ _ w249 w256 w262 w267 w272]
      tunnel: [_ _ _ "停止" _ _ _] -> w227
      tunnel: w226 -> [_ _ _ w253 _ _ _]
      event Timeout {
        n106 = event-data() -> ()  [unwired: 1 in, 3 out]
      }
      event "VISA Resource": Value Change {
        n107 = event-data() -> ()  [unwired: 1 in, 6 out]
        n108 = call <vilib>:"Application Directory.vi"() -> ("Application Directory"=w231:path)
        n109 = Build Path(base path=w231, name or relative path="data\\set.ini" ("名称或相对路径")) -> (appended path=w232:path)
        n110 = call <vilib>:"Open Config Data.vi"("configuration file path"=w232) -> ("error out"=w238:errorcluster, "refnum"=w237:T8)  [unwired: 8 in, 1 out]
        n111 = call-poly <vilib>:"Write Key.vi"("section"="CODMn", "error in (no error)"=w238, "value"="VISA Resource", "key"="串口", "refnum"=w237) -> ("error out"=w234:errorcluster, "refnum out"=w230:T8)  [unwired: 4 in, 1 out]
        n112 = call <vilib>:"Close Config Data.vi"("error in (no error)"=w234, "refnum"=w230) -> ()  [unwired: 8 in, 2 out]
      }
      event "启动": Value Change {
        n113 = event-data() -> ()  [unwired: 1 in, 6 out]
        n114 = case shown="默认" "控制命令" {
          tunnel: "控制命令参数" -> [w251 w252]
          tunnel: [w250 w252] -> w239
          frame Default {
            n115 = call "HexToWord.vi"("数组"=w251) -> ("WORD"=w250:u16[])  [unwired: 10 in]
          }
          frame 13 {
          }
        }
        n116 = Swap Bytes(anything="控制命令") -> (byte swapped=w242:u16)
        n117 = call "控制命令区.vi"("控制命令参数"=w239, "控制命令"=w242) -> ("控制命令"=w245:u16[])  [unwired: 9 in]
        n118 = local read "站号"() -> (w244:u16)
        n119 = Bundle("站号"=w244, "控制命令"=w245) -> (w243:cluster{"站号":u16, "控制命令":u16[]})  [unwired: 1 in]
        n120 = Bundle By Name(cluster=cluster{"命令":string, "data":variant} {"命令"="", "data"=variant} ("元素"), "命令"="启动", "data"=w243) -> (w247:cluster{"命令":string, "data":variant})
        n121 = Enqueue Element(queue=w249, element=w247) -> ()  [unwired: 2 in, 3 out]
      }
      event "停止": Value Change {
        n122 = event-data() -> ()  [unwired: 1 in, 6 out]
        n123 = Set Occurrence(w253) -> ()
        n124 = Flush Queue(queue=w256) -> (queue out=w255:refnum<queue>)  [unwired: 1 in, 2 out]
        n125 = Enqueue Element(queue=w255, element=cluster{"命令":string, "data":variant} {"命令"="shutdown", "data"=variant} ("元素")) -> ()  [unwired: 2 in, 3 out]
      }
      event "读测量数据区": Value Change {
        n126 = event-data() -> ()  [unwired: 1 in, 6 out]
        n127 = Bundle By Name(cluster=cluster{"命令":string, "data":variant} {"命令"="", "data"=variant} ("元素"), "命令"="读测量数据区", "data"="站号") -> (w260:cluster{"命令":string, "data":variant})
        n128 = Enqueue Element(queue=w262, element=w260) -> ()  [unwired: 2 in, 3 out]
      }
      event "读状态告警区": Value Change {
        n129 = event-data() -> ()  [unwired: 1 in, 6 out]
        n130 = local read "站号"() -> (w263:u16)
        n131 = Bundle By Name(cluster=cluster{"命令":string, "data":variant} {"命令"="", "data"=variant} ("元素"), "命令"="读状态告警区", "data"=w263) -> (w265:cluster{"命令":string, "data":variant})
        n132 = Enqueue Element(queue=w267, element=w265) -> ()  [unwired: 2 in, 3 out]
      }
      event "读关键参数区": Value Change {
        n133 = event-data() -> ()  [unwired: 1 in, 6 out]
        n134 = local read "站号"() -> (w268:u16)
        n135 = Bundle By Name(cluster=cluster{"命令":string, "data":variant} {"命令"="", "data"=variant} ("元素"), "命令"="读关键参数区", "data"=w268) -> (w270:cluster{"命令":string, "data":variant})
        n136 = Enqueue Element(queue=w272, element=w270) -> ()  [unwired: 2 in, 3 out]
      }
    }
  }
  n137 = while "While循环" {
    tunnel: w21 -> [w275]
    tunnel: w27 -> [w274]
    stop <- FALSE stop-if-true
    # "TCP掉线重连"
    n138 = global read "CODMn断电保存全局变量.vi" "MB通信方式选择"() -> (w273:enum16{"串口", "TCP"})
    n139 = Wait (ms)(milliseconds to wait=u32 10000 ("等待时间（毫秒）")) -> ()  [unwired: 1 out]
    n140 = case shown="\"TCP\"" w273 {
      tunnel: w275 -> [_ w280]
      tunnel: w274 -> [_ w279]
      frame "串口", Default {
      }
      frame "TCP" {
        n141 = global read "VARCODMn全局变量.vi" "MB session in"() -> (w278:refnum<class "MB_Master.lvclass">)
        n142 = property class="MB_Master"(reference=w278) -> ("Properties:Session Valid"=w281:bool)  [unwired: 1 in, 2 out]
        n143 = case shown="假" w281 {
          tunnel: w280 -> [w284 _]
          tunnel: w279 -> [w283 _]
          frame False {
            n144 = Flush Queue(queue=w284, error in (no error)=w283) -> (queue out=w286:refnum<queue>, error out=w285:errorcluster)  [unwired: 1 out]
            n145 = Enqueue Element(queue=w286, element=cluster{"命令":string, "data":variant} {"命令"="启用模块", "data"=variant} ("元素"), error in (no error)=w285) -> ()  [unwired: 1 in, 3 out]
          }
          frame True {
          }
        }
      }
    }
  }
  n146 = call "反控参数变更.vi"("设置参数"=T4."CODMn") -> ()  [unwired: 11 in]
  n147 = while {
    tunnel: w21 -> [w301]
    tunnel: w27 -> [w300]
    shift-right: [w298] -> _
    shift-left: _ -> [w297]
    tunnel: errorcluster {"status"=FALSE, "code"=0, "source"=""} ("error out") -> [w296]
    tunnel: [w291] -> _
    tunnel: w29 -> [_]
    stop <- w299 stop-if-true
    n148 = Dequeue Element(queue=w301, error in (no error)=w300) -> (queue out=w292:refnum<queue>, element=w294:cluster{"命令":string, "data":variant})  [unwired: 1 in, 2 out]
    n149 = Unbundle By Name(w294) -> ("命令"=w295:string, "data"=w293:variant)
    n150 = case shown="\"读状态告警区\"" w295 {
      tunnel: w293 -> [_ _ _ w328 w339 w356 w368 w377 w387 w415 w430 w450 _]
      tunnel: w292 -> [_ _ _ _ _ _ _ _ _ _ _ _ w505]
      tunnel: [_ _ _ _ _ _ _ _ _ _ _ _ TRUE] -> w299
      tunnel: [w310 w313 w315 w331 w342 w358 w370 w382 w396 w422 w437 w445 w501] -> w298
      tunnel: [w311 w312 w316 w330 w341 w357 w369 w371 w385 w411 w438 w444 w502] -> w291
      tunnel: w297 -> [w310 _ w315 w327 w338 w355 w367 w376 w390 w418 w433 w451 w501]
      tunnel: w296 -> [w311 _ w318 w324 w335 w352 w364 w374 w391 w419 w434 w452 w503]
      frame Default {
      }
      frame "启用模块" {
        n151 = call "MB_api.vi"("STEP"=enum16{"open", "read", "write", "close"}."open") -> ("error out"=w312:errorcluster, "MB session out"=w313:refnum<class "MB_Master.lvclass">)  [unwired: 8 in, 1 out]
        n152 = global write "VARCODMn全局变量.vi" "MB session in"(w313) -> ()
      }
      frame "停用模块" {
        n153 = call-dynamic "Close Session.vi"("error in (no error)"=w318, "MB session in"=w315) -> ("error out"=w317:errorcluster)  [unwired: 9 in]
        n154 = call <vilib>:"Clear Errors.vi"("error in (no error)"=w317) -> ("error out"=w316:errorcluster)  [unwired: 5 in, 1 out]
      }
      frame "启动" {
        n155 = Variant To Data(type=cluster{"站号":u16, "控制命令":u16[]} {"站号"=0, "控制命令"=[]} ("输出簇"), Variant=w328) -> (data=w322:cluster{"站号":u16, "控制命令":u16[]})  [unwired: 1 in, 1 out]
        n156 = Unbundle By Name(w322) -> ("站号"=w321:u16, "控制命令"=w319:u16[])
        n157 = property class="MB_Master"(reference=w327, error in=w324, "Properties:Slave ID"=w321) -> (reference out=w326:refnum<class "MB_Master.lvclass">, error out=w325:errorcluster)
        n158 = Index Array(array=w319) -> (element=w320:u16)  [unwired: 1 in]
        n159 = global write "VARCODMn全局变量.vi" "控制命令"(w320) -> ()
        n160 = call <vilib>:"Write Multiple Registers.vi"("error in (no error)"=w325, "values"=w319, "starting address"=u16 4608, "MB session in"=w326) -> ("error out"=w330:errorcluster, "MB session out"=w331:refnum<class "MB_Master.lvclass">)  [unwired: 6 in]
      }
      frame "盲样测试" {
        n161 = Variant To Data(type=0, Variant=w339) -> (data=w332:i32)  [unwired: 1 in, 1 out]
        n162 = property class="MB_Master"(reference=w338, error in=w335, "Properties:Slave ID"=w332) -> (reference out=w337:refnum<class "MB_Master.lvclass">, error out=w336:errorcluster)
        n163 = case shown="默认" w332 {
          tunnel: [u16[] [] ("values") u16[] [33539, 0] ("values") u16[] [23555, 0] ("values")] -> w334
          frame Default {
          }
          frame 1 {
            # "总磷盲样测试命令"
          }
          frame 3 {
            # "氨氮盲样测试"
          }
        }
        n164 = call <vilib>:"Write Multiple Registers.vi"("error in (no error)"=w336, "values"=w334, "starting address"=u16 24592, "MB session in"=w337) -> ("error out"=w341:errorcluster, "MB session out"=w342:refnum<class "MB_Master.lvclass">)  [unwired: 6 in]
      }
      frame "debug" {
        n165 = Variant To Data(type=cluster{"站号":u16, "控制命令":u16[]} {"站号"=0, "控制命令"=[]} ("输出簇"), Variant=w356) -> (data=w350:cluster{"站号":u16, "控制命令":u16[]})  [unwired: 1 in, 1 out]
        n166 = Unbundle By Name(w350) -> ("站号"=w349:u16, "控制命令"=w347:u16[])
        "控制命令 2" <- w347
        n167 = property class="MB_Master"(reference=w355, error in=w352, "Properties:Slave ID"=w349) -> (reference out=w354:refnum<class "MB_Master.lvclass">, error out=w353:errorcluster)
        n168 = Index Array(array=w347) -> (element=w348:u16)  [unwired: 1 in]
        n169 = global write "VARCODMn全局变量.vi" "控制命令"(w348) -> ()
        n170 = call <vilib>:"Write Multiple Registers.vi"("error in (no error)"=w353, "values"=w347, "starting address"=u16 24594, "MB session in"=w354) -> ("error out"=w357:errorcluster, "MB session out"=w358:refnum<class "MB_Master.lvclass">)  [unwired: 6 in]
      }
      frame "单步控制" {
        n171 = Variant To Data(type=cluster{"站号":u16, "控制命令":u16[]} {"站号"=0, "控制命令"=[]} ("输出簇"), Variant=w368) -> (data=w362:cluster{"站号":u16, "控制命令":u16[]})  [unwired: 1 in, 1 out]
        n172 = Unbundle By Name(w362) -> ("站号"=w361:u16, "控制命令"=w360:u16[])
        n173 = property class="MB_Master"(reference=w367, error in=w364, "Properties:Slave ID"=w361) -> (reference out=w366:refnum<class "MB_Master.lvclass">, error out=w365:errorcluster)
        n174 = call <vilib>:"Write Multiple Registers.vi"("error in (no error)"=w365, "values"=w360, "starting address"=u16 24610, "MB session in"=w366) -> ("error out"=w369:errorcluster, "MB session out"=w370:refnum<class "MB_Master.lvclass">)  [unwired: 6 in]
      }
      frame "读测量数据区" {
        n175 = Variant To Data(type=u8 1 ("Slave ID"), Variant=w377) -> (data=w378:u8)  [unwired: 1 in, 1 out]
        n176 = property class="MB_Master"(reference=w376, error in=w374, "Properties:Slave ID"=w378) -> (reference out=w375:refnum<class "MB_Master.lvclass">, error out=w373:errorcluster)
        n177 = call <vilib>:"Read Holding Registers.vi"("error in (no error)"=w373, "quantity"=u16 105, "starting address"=u16 4096, "MB session in"=w375) -> ("error out"=w371:errorcluster, "Registers"=w372:u16[], "MB session out"=w382:refnum<class "MB_Master.lvclass">)  [unwired: 5 in]
        n178 = case shown="无错误" w371 {
          tunnel: w372 -> [w384 _]
          frame No Error {
            n179 = call "测量数据区.vi"("数组"=w384) -> ("测量数据区"=w383:T2)  [unwired: 10 in]
            "测量数据区" <- w383
            n180 = global write "VARCODMn全局变量.vi" "测量数据区"(w383) -> ()
            "测量数据区" <- w384
          }
          frame Error {
          }
        }
      }
      frame "读状态告警区" {
        n181 = Variant To Data(type=u8 1 ("Slave ID"), Variant=w387) -> (data=w392:u8)  [unwired: 1 in, 1 out]
        n182 = property class="MB_Master"(reference=w390, error in=w391, "Properties:Slave ID"=w392) -> (reference out=w389:refnum<class "MB_Master.lvclass">, error out=w388:errorcluster)
        n183 = call <vilib>:"Read Holding Registers.vi"("error in (no error)"=w388, "quantity"=u16 56, "starting address"=u16 4224, "MB session in"=w389) -> ("error out"=w385:errorcluster, "Registers"=w386:u16[], "MB session out"=w396:refnum<class "MB_Master.lvclass">)  [unwired: 5 in]
        n184 = case shown="无错误" w385 {
          tunnel: w386 -> [w410 _]
          frame No Error {
            n185 = call "状态告警区.vi"("数组"=w410) -> ("状态告警区"=w407:T1)  [unwired: 10 in]
            "状态告警区" <- w407
            n186 = global write "VARCODMn全局变量.vi" "状态告警区"(w407) -> ()
            n187 = Unbundle By Name(w407) -> ("A"=w400:sgl, "B"=w399:sgl, "K"=w398:sgl, "光值1"=w406:sgl, "光值2"=w405:sgl, "光值3"=w404:sgl, "光值4"=w403:sgl, "光值5"=w402:sgl, "光值6"=w401:sgl)
            n188 = global read "工况数据接口全局.vi" "data"() -> (w408:T17)
            n189 = Bundle By Name(cluster=w408, "data.CODMn.CODMn.F0"=w406, "data.CODMn.CODMn.F1"=w405, "data.CODMn.CODMn.F2"=w404, "data.CODMn.CODMn.F3"=w403, "data.CODMn.CODMn.F4"=w402, "data.CODMn.CODMn.F5"=w401, "data.CODMn.CODMn.A"=w400, "data.CODMn.CODMn.B"=w399, "data.CODMn.CODMn.K"=w398, "data.CODMn.启用"=TRUE) -> (w409:T17)
            n190 = global write "工况数据接口全局.vi" "data"(w409) -> ()
            "状态告警区" <- w410
          }
          frame Error {
          }
        }
      }
      frame "读关键参数区" {
        n191 = Variant To Data(type=u8 1 ("Slave ID"), Variant=w415) -> (data=w413:u8)  [unwired: 1 in, 1 out]
        n192 = property class="MB_Master"(reference=w418, error in=w419, "Properties:Slave ID"=w413) -> (reference out=w417:refnum<class "MB_Master.lvclass">, error out=w416:errorcluster)
        n193 = call <vilib>:"Read Holding Registers.vi"("error in (no error)"=w416, "quantity"=u16 19, "starting address"=u16 4256, "MB session in"=w417) -> ("error out"=w411:errorcluster, "Registers"=w412:u16[], "MB session out"=w422:refnum<class "MB_Master.lvclass">)  [unwired: 5 in]
        n194 = case shown="无错误" w411 {
          tunnel: w412 -> [w424 _]
          frame No Error {
            n195 = call "关键参数区.vi"("数组"=w424) -> ("关键参数区"=w423:T3)  [unwired: 10 in]
            "关键参数区" <- w423
            n196 = global write "VARCODMn全局变量.vi" "关键参数区"(w423) -> ()
          }
          frame Error {
          }
        }
      }
      frame "读序列号" {
        n197 = Variant To Data(type=u8 1 ("Slave ID"), Variant=w430) -> (data=w428:u8)  [unwired: 1 in, 1 out]
        n198 = property class="MB_Master"(reference=w433, error in=w434, "Properties:Slave ID"=w428) -> (reference out=w432:refnum<class "MB_Master.lvclass">, error out=w431:errorcluster)
        n199 = call <vilib>:"Read Holding Registers.vi"("error in (no error)"=w431, "quantity"=u16 6, "starting address"=u16 4, "MB session in"=w432) -> ("error out"=w438:errorcluster, "Registers"=w427:u16[], "MB session out"=w437:refnum<class "MB_Master.lvclass">)  [unwired: 5 in]
        n200 = call "HexToString.vi"("数组"=w427) -> ("STRING"=w426:string[])  [unwired: 10 in]
        n201 = Index Array(array=w426) -> (element=w425:string)  [unwired: 1 in]
        "序列号" <- w425
        n202 = global write "VARCODMn全局变量.vi" "序列号"(w425) -> ()
      }
      frame "读滴定曲线" {
        n203 = Variant To Data(type=u8 1 ("Slave ID"), Variant=w450) -> (data=w448:u8)  [unwired: 1 in, 1 out]
        n204 = property class="MB_Master"(reference=w451, error in=w452, "Properties:Slave ID"=w448) -> (reference out=w447:refnum<class "MB_Master.lvclass">, error out=w446:errorcluster)
        n205 = global read "VARCODMn全局变量.vi" "固件版本"() -> (w443:cluster{"V5以上版本":bool, "版本号":dbl})
        n206 = Unbundle By Name(w443) -> ("V5以上版本"=w442:bool)
        n207 = case shown="真" w442 {
          tunnel: w447 -> [w456 w481]
          tunnel: w446 -> [w457 w480]
          tunnel: [w453 w479] -> w439
          tunnel: [w455 w478] -> w445
          tunnel: [w454 w477] -> w444
          frame False {
            n208 = for {
              tunnel: u16[] [120, 120, 120, 120, 32] -> [w472] mode=indexing
              shift-right: [w476] -> _
              shift-left: u16 24599 ("starting address") -> [w473]
              shift-right: [w474] -> w458
              shift-left: u16[] [] ("新元素/子数组") -> [w475]
              tunnel: w456 -> [w471]
              tunnel: w457 -> [w470]
              tunnel: [w469] -> w455
              tunnel: [w468] -> w454
              n209 = Add(x=w473, y=w472) -> (x+y=w476:u16)
              n210 = call <vilib>:"Read Holding Registers.vi"("error in (no error)"=w470, "quantity"=w472, "starting address"=w473, "MB session in"=w471) -> ("error out"=w468:errorcluster, "Registers"=w467:u16[], "MB session out"=w469:refnum<class "MB_Master.lvclass">)  [unwired: 5 in]
              n211 = call "HexToWord.vi"("数组"=w467) -> ("WORD"=w466:u16[])  [unwired: 10 in]
              n212 = Insert Into Array(array=w475, new element=w466) -> (w474:u16[])  [unwired: 1 in]
            }
            n213 = for {
              tunnel: w458 -> [w465] mode=indexing
              tunnel: [w462] -> w453 mode=indexing
              n214 = Divide(x=w465, y=u16 10) -> (x/y=w463:dbl)
              n215 = To Unsigned Word Integer(number=w463) -> (unsigned 16bit integer=w462:u16)
            }
          }
          frame True {
            n216 = for {
              tunnel: u16[] [120, 120, 120, 120, 32] -> [w496] mode=indexing
              shift-right: [w500] -> _
              shift-left: u16 24615 ("starting address") -> [w497]
              shift-right: [w498] -> w482
              shift-left: u16[] [] ("新元素/子数组") -> [w499]
              tunnel: w481 -> [w495]
              tunnel: w480 -> [w494]
              tunnel: [w493] -> w478
              tunnel: [w492] -> w477
              n217 = Add(x=w497, y=w496) -> (x+y=w500:u16)
              n218 = call <vilib>:"Read Holding Registers.vi"("error in (no error)"=w494, "quantity"=w496, "starting address"=w497, "MB session in"=w495) -> ("error out"=w492:errorcluster, "Registers"=w491:u16[], "MB session out"=w493:refnum<class "MB_Master.lvclass">)  [unwired: 5 in]
              n219 = call "HexToWord.vi"("数组"=w491) -> ("WORD"=w490:u16[])  [unwired: 10 in]
              n220 = Insert Into Array(array=w499, new element=w490) -> (w498:u16[])  [unwired: 1 in]
            }
            n221 = for {
              tunnel: w482 -> [w489] mode=indexing
              tunnel: [w486] -> w479 mode=indexing
              n222 = Divide(x=w489, y=u16 5) -> (x/y=w487:dbl)
              n223 = To Unsigned Word Integer(number=w487) -> (unsigned 16bit integer=w486:u16)
            }
          }
        }
        n224 = global write "VARCODMn全局变量.vi" "滴定数-ORP值"(w439) -> ()
        n225 = global read "工况数据接口全局.vi" "data"() -> (w440:T17)
        n226 = global write "VARCODMn全局变量.vi" "ORP滴定曲线"(w439) -> ()
        n227 = Bundle By Name(cluster=w440, "data.CODMn.CODMn.titration_curve"=w439) -> (w441:T17)
        n228 = global write "工况数据接口全局.vi" "data"(w441) -> ()
      }
      frame "shutdown" {
        n229 = call-dynamic "Close Session.vi"("error in (no error)"=w503, "MB session in"=w501) -> ("error out"=w502:errorcluster)  [unwired: 9 in]
        n230 = Flush Queue(queue=w505) -> (queue out=w504:refnum<queue>)  [unwired: 1 in, 2 out]
        n231 = Release Queue(queue=w504) -> ()  [unwired: 2 in, 3 out]
      }
    }
    n232 = Unbundle By Name(w291) -> ("status"=w287:bool)
    n233 = call <vilib>:"Boolean Crossing PtByPt.vi"("direction"=enum16{"either", "false-true", "true-false"}."either", "input"=w287) -> ("crossing"=w288:bool)  [unwired: 1 in]
    n234 = Not(x=w287) -> (.not. x?=w290:bool)
    "status" <- w290
    n235 = global write "VARCODMn全局变量.vi" "通讯状态"(w290) -> ()
    n236 = case shown="真" w288 {
      tunnel: w287 -> [_ w305]
      frame False {
      }
      frame True {
        n237 = case shown="真" w305 {
          tunnel: ["0" "999"] -> w304
          frame False {
          }
          frame True {
          }
        }
        n238 = Bundle By Name(cluster=T16 {"name"="", "CN"="", "FirmwareVersion"="", "code"=""} ("map in"), "name"="CODMn" ("componentParent"), "FirmwareVersion"="V3" ("equipVersion"), "code"=w304) -> (w302:T16)
        n239 = call "告警接口-告警存储-交互.vi"("map in"=w302) -> ()  [unwired: 10 in, 1 out]
      }
    }
  }
  n240 = Release Queue(queue=w3, error in (no error)=w2) -> ()  [unwired: 1 in, 3 out]
  n241 = Release Queue(queue=w20, error in (no error)=w19) -> ()  [unwired: 1 in, 3 out]
  n242 = Release Queue(queue=w13, error in (no error)=w12) -> ()  [unwired: 1 in, 3 out]
